vi "SaveConfigGUI.vi"(4 "error in (no error)":errorcluster, 6 "Current Configuration":T1 {"Select Mode:" items=["Custom", "Imaging", "300 All", "600 UV", "600 Blue", "600 Mid", "600 Red", "1200 m0", "1200 m1", "1200 m2", "1200 m3", "1200 m4", "1200 m5", "1200 m6", "1200 m7", "1200 RESOLVE", "400 m1", "400 m2", "930 m1", "930 m2", "930 m3", "930 m4", "930 m5", "930 m6", "400KL"]}) -> (0 "error out":errorcluster, 1 "Canceled?":bool, 2 "Configuration Written":T1 {"Select Mode:" items=["Custom", "Imaging", "300 All", "600 UV", "600 Blue", "600 Mid", "600 Red", "1200 m0", "1200 m1", "1200 m2", "1200 m3", "1200 m4", "1200 m5", "1200 m6", "1200 m7", "1200 RESOLVE", "400 m1", "400 m2", "930 m1", "930 m2", "930 m3", "930 m4", "930 m5", "930 m6", "400KL"]})   [LabVIEW 2015]
uses:
  GSCS Scripting/GSCS-Scripting/Utils/GSP_ObsConfig.llb/configuration.ctl
  GSP_GUI_global.vi
panel:
  in  "Config Details":i32(listbox)
  in  "Save":bool
  in  "Configuration Name":string="default"
  # "The configuration file will be written\nto your user directory"
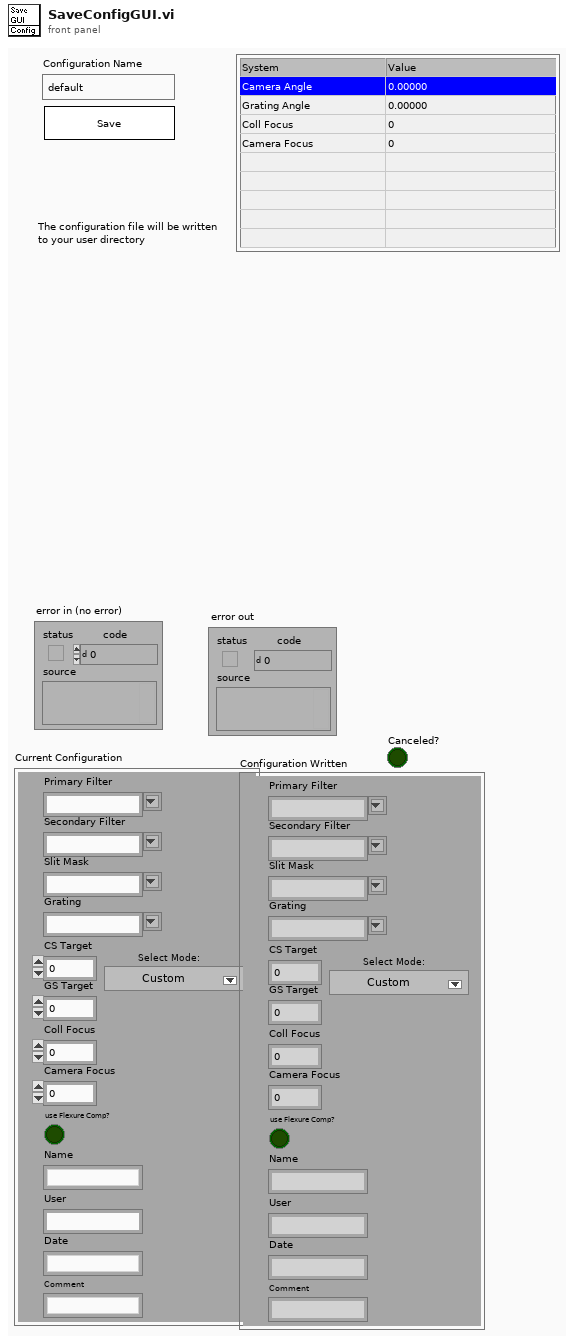
[diagram p1: front panel]
types:
  T1 = typedef "configuration.ctl" = cluster{"Primary Filter":string, "Secondary Filter":string, "Slit Mask":string, "Grating":string, "CS Target":dbl, "GS Target":dbl, "Coll Focus":i32, "Camera Focus":i32, "Name":string, "User":string, "Date":string, "Comment":string, "use Flexure Comp?":bool, "Select Mode:":u16}
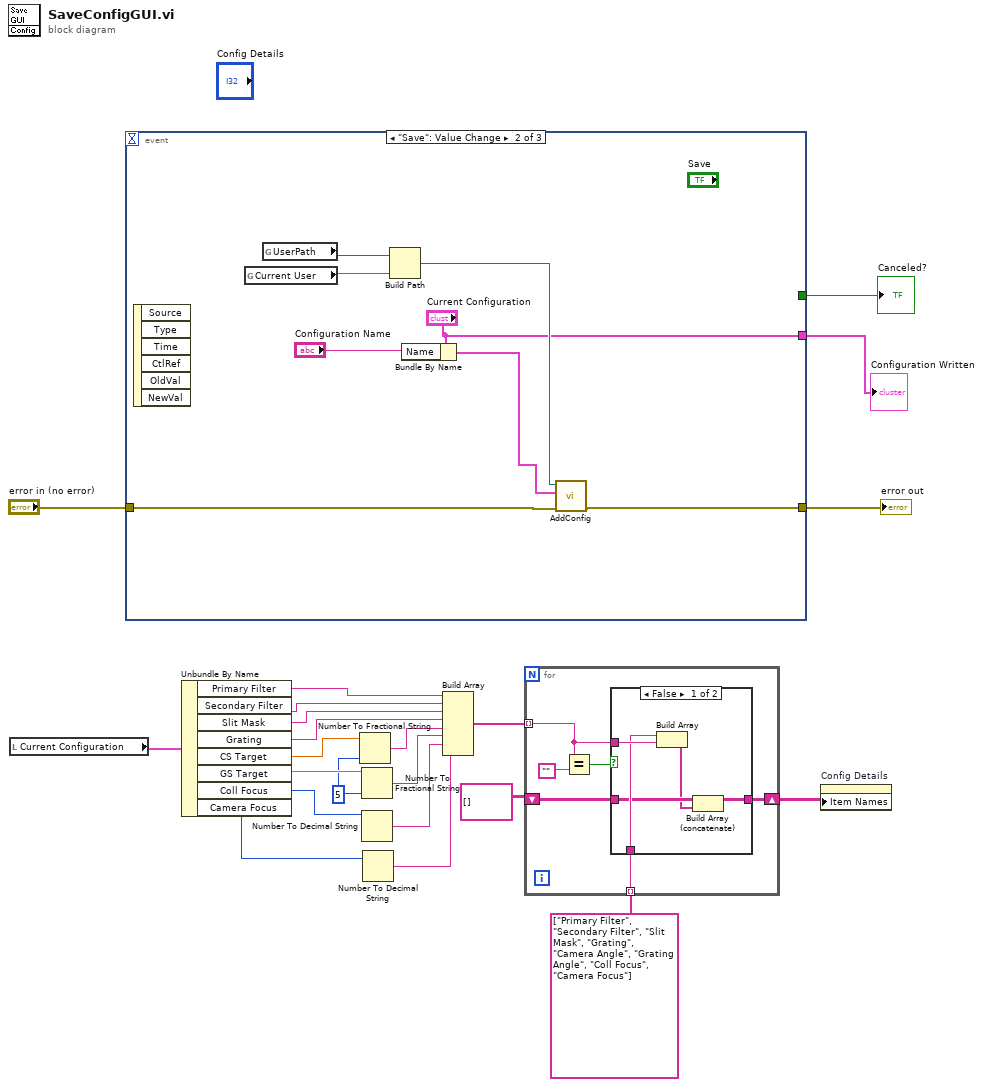
[diagram p0: block diagram]
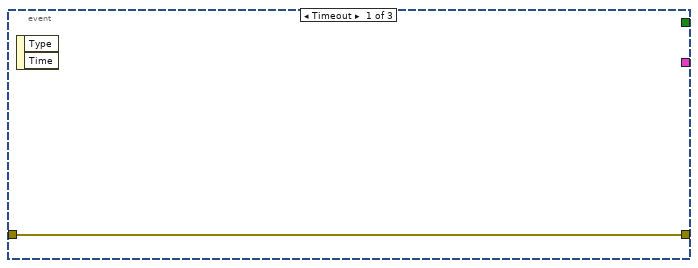
[diagram p3: hidden frame]
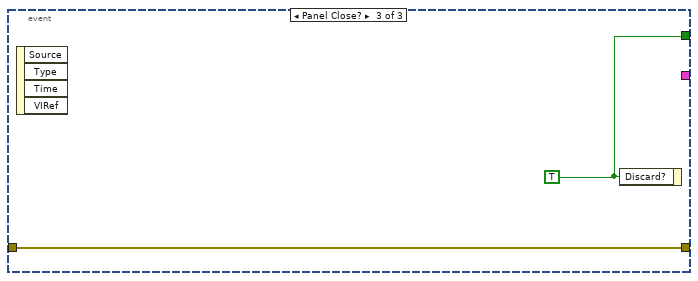
[diagram p4: hidden frame]
diagram:
  w8 = 5
  n1 = local read "Current Configuration"() -> (w19:T1)
  n2 = event shown="[1] \"Save\": Value Change" {
    selector: _ -> [_ _ _]
    dyn-events: _ -> [_ _ _]
    timeout: _ -> [_ _ _]
    tunnel: [_ _ w32] -> w20
    tunnel: "error in (no error)" -> [w23 w28 w33]
    tunnel: [w23 w27 w33] -> w21
    tunnel: [_ "Current Configuration" _] -> w1
    event Timeout {
      n3 = event-data() -> ()  [unwired: 1 in, 2 out]
    }
    event "Save": Value Change {
      n4 = event-data() -> ()  [unwired: 1 in, 6 out]
      n5 = global read "GSP_GUI_global.vi" "Current User"() -> (w30:string)
      n6 = global read "GSP_GUI_global.vi" "UserPath"() -> (w31:path)
      n7 = Build Path(base path=w31, name or relative path=w30) -> (appended path=w26:path)
      n8 = Bundle By Name(cluster="Current Configuration", "Name"="Configuration Name") -> (w25:T1)
      n9 = call "AddConfig.vi"("error in (no error)"=w28, "Configuration In"=w25, "path"=w26) -> ("error out"=w27:errorcluster)  [unwired: 4 in]
    }
    event Panel Close? {
      w32 = TRUE
      n10 = event-data() -> ()  [unwired: 1 in, 4 out]
      n11 = event-data("Discard?"=w32) -> ()  [unwired: 1 in, 1 out]
    }
  }
  "error out" <- w21
  "Canceled?" <- w20
  "Configuration Written" <- w1
  n12 = Unbundle By Name(w19) -> ("Primary Filter"=w18:string, "Secondary Filter"=w17:string, "Slit Mask"=w6:string, "Grating"=w7:string, "CS Target"=w16:dbl, "GS Target"=w14:dbl, "Coll Focus"=w12:i32, "Camera Focus"=w11:i32)
  n13 = Number To Fractional String(number=w16, precision (6)=w8) -> (F-format string=w15:string)  [unwired: 2 in]
  n14 = Number To Fractional String(number=w14, precision (6)=w8) -> (F-format string=w13:string)  [unwired: 2 in]
  n15 = Number To Decimal String(number=w12) -> (decimal integer string=w10:string)  [unwired: 1 in]
  n16 = Number To Decimal String(number=w11) -> (decimal integer string=w9:string)  [unwired: 1 in]
  n17 = Build Array(w18, w17, w6, w7, w15, w13, w10, w9) -> (w5:string[])
  n18 = for {
    tunnel: w5 -> [w36] mode=indexing
    tunnel: string[] ["Primary Filter", "Secondary Filter", "Slit Mask", "Grating", "Camera Angle", "Grating Angle", "Coll Focus", "Camera Focus"] -> [w35] mode=indexing
    shift-right: [w34] -> w2
    shift-left: string[][] [] -> [w37]
    n19 = Equal?(x=w36, y="") -> (x = y?=w38:bool)
    n20 = case shown="False" w38 {
      tunnel: w37 -> [w42 w45]
      tunnel: w36 -> [w44 _]
      tunnel: w35 -> [w43 _]
      tunnel: [w40 w45] -> w34
      frame False {
        n21 = Build Array(w43, w44) -> (w41:string[])
        n22 = Build Array (concatenate)(w42, w41) -> (w40:string[][])
      }
      frame True {
      }
    }
  }
  n23 = property on="Config Details" class="MCListbox (strict)"("Item Names"=w2) -> ()  [unwired: 2 in, 2 out]
